vi "Configure Jitter Spectrum (Data Rate-Unit Interval).vi"(0 "VISA resource name":refnum<visa-resource-name>, 1 "Enable Jitter Spectrum (Enable)":bool, 5 "Channel (1: Channel 1)":i32(ring) items=["Channel 1", "Channel 2", "Channel 3", "Channel 4", "Function 1", "Function 2", "Function 3", "Function 4", "Memory 1", "Memory 2", "Memory 3", "Memory 4"], 7 "Measurement (0: Data Rate)":i32(ring) items=["Data Rate", "Unit Interval"], 9 "Data Rate Type (0: Fully Automatic)":i32(ring) items=["Fully Automatic", "Semi Automatic"], 11 "error in (no error)":errorcluster, 12 "Data Rate (2.5E9 Hz)":dbl) -> (4 "VISA resource name out":refnum<visa-resource-name>, 15 "error out":errorcluster)   [LabVIEW 2009, in "Agilent 8000 Series.lvlib"]
doc: "Configures the Data Rate or Unit Interval measurement and enables the Jitter Spectrum Jitter analysis on it.\n\n<B>Note:</B>\nCalling this VI disables all previously enabled measurements and clears existing measurement results from display."
uses:
  Agilent 8000 Series.lvlib
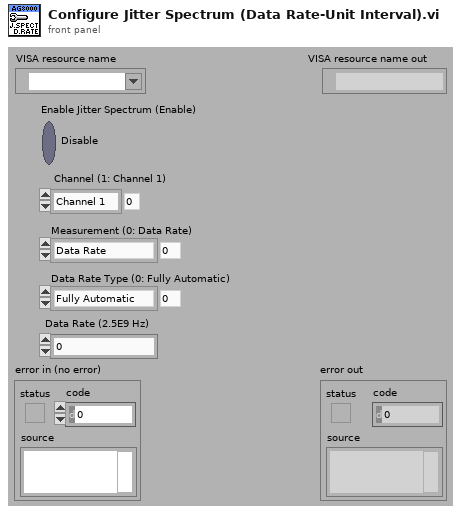
[diagram p1: front panel]
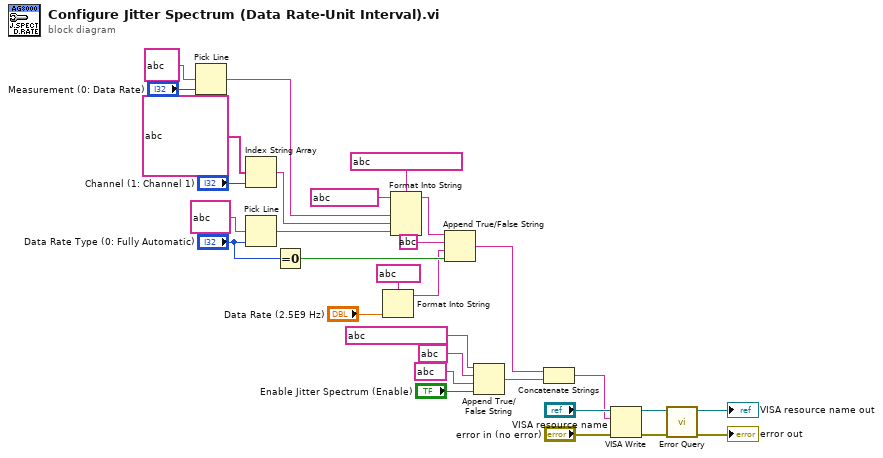
[diagram p0: block diagram]
diagram:
  n1 = Pick Line(multi-line string=string ?, line index="Measurement (0: Data Rate)") -> (output string=w1:string)  [unwired: 1 in]
  n2 = Index String Array(1:"Channel (1: Channel 1)", 2:string[] ?) -> (0:w2:string)  [unwired: 1 in]
  n3 = Pick Line(multi-line string=string ?, line index="Data Rate Type (0: Fully Automatic)") -> (output string=w9:string)  [unwired: 1 in]
  n4 = Equal To 0?(x="Data Rate Type (0: Fully Automatic)") -> (x = 0?=w13:bool)
  n5 = Format Into String(format string=string ?, "Data Rate (2.5E9 Hz)") -> (resulting string=w8:string)  [unwired: 2 in, 1 out]
  n6 = Format Into String(format string=string ?, initial string=string ? ("format string"), w1, w2, w9) -> (resulting string=w7:string)  [unwired: 1 in, 1 out]
  n7 = Append True/False String(1:w13, 2:w8, 3:string ?, 4:w7) -> (0:w6:string)
  n8 = Append True/False String(1:"Enable Jitter Spectrum (Enable)", 2:string ? ("false string"), 3:string ? ("true string"), 4:string ? ("string (\"\")")) -> (0:w15:string)
  n9 = Concatenate Strings(w6, w15) -> (w16:string)
  n10 = VISA Write(VISA resource name="VISA resource name", write buffer=w16, error in (no error)="error in (no error)") -> (VISA resource name out=w26:refnum<visa-resource-name>, error out=w25:errorcluster)  [unwired: 1 out]
  n11 = call "Error Query.vi"("error in (no error)"=w25, "VISA resource name"=w26) -> ("error out"=→"error out":errorcluster, "VISA resource name out"=→"VISA resource name out":refnum<visa-resource-name>)  [unwired: 6 in, 2 out]
